vi "Q-Insert.vi"(6 "timeout in ms (-1)":i32=-1, 7 "Queue Type":T1, 8 "error in":errorcluster, 9 "Index":i32, 10 "Read Data":T2, 11 "Q Name":string) -> (0 "error out":errorcluster)   [LabVIEW 2016]
uses:
  PSDAQEG_Task Queue Type.ctl
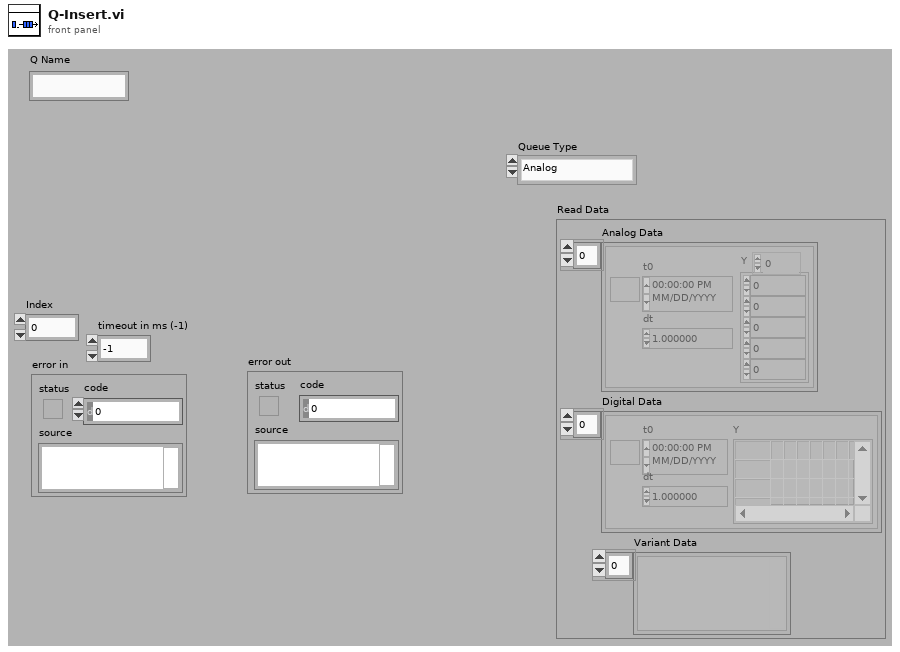
[diagram p1: front panel]
types:
  T1 = typedef "PSDAQEG_Task Queue Type.ctl" = enum16{"Analog", "Digital", "Variant"}
  T2 = cluster{"Analog Data":waveform(dbl)[], "Digital Data":digitalwaveform[], "Variant Data":variant[]}
  T3 = cluster{"Index":i32, "Analog Data":waveform(dbl)[]}
  T4 = cluster{"Index":i32, "Digital Data":digitalwaveform[]}
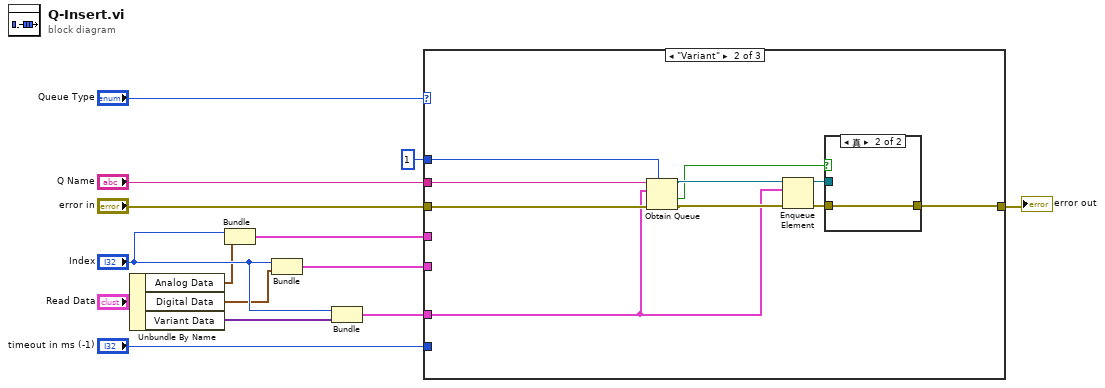
[diagram p0: block diagram]
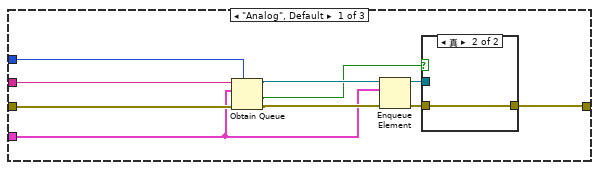
[diagram p2: hidden frame]
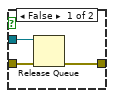
[diagram p3: hidden frame]
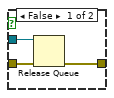
[diagram p4: hidden frame]
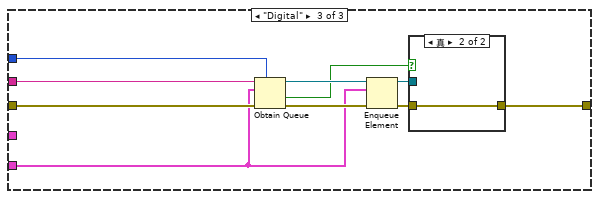
[diagram p5: hidden frame]
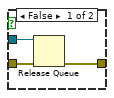
[diagram p6: hidden frame]
diagram:
  n1 = Unbundle By Name("Read Data") -> ("Analog Data"=w1:waveform(dbl)[], "Digital Data"=w3:digitalwaveform[], "Variant Data"=w2:variant[])
  n2 = Bundle("Index"="Index", "Analog Data"=w1) -> (w12:T3)  [unwired: 1 in]
  n3 = Bundle("Index"="Index", "Digital Data"=w3) -> (w13:T4)  [unwired: 1 in]
  n4 = Bundle("Index"="Index", "Variant Data"=w2) -> (w11:cluster{"Index":i32, "Variant Data":variant[]})  [unwired: 1 in]
  n5 = case shown="\"Variant\"" "Queue Type" {
    tunnel: "Q Name" -> [w23 w37 w52]
    tunnel: "error in" -> [w24 w38 w51]
    tunnel: 1 ("Index") -> [w22 w36 w50]
    tunnel: w13 -> [_ _ w43]
    tunnel: [w18 w31 w46] -> w10
    tunnel: w12 -> [w17 _ _]
    tunnel: w11 -> [_ w29 _]
    tunnel: "timeout in ms (-1)" -> [_ _ _]
    frame "Analog", Default {
      n6 = Obtain Queue(max queue size (-1, unlimited)=w22, name (unnamed)=w23, element data type=w17, error in (no error)=w24) -> (queue out=w16:refnum<queue>, created new?=w15:bool, error out=w19:errorcluster)  [unwired: 1 in]
      n7 = Enqueue Element(queue=w16, element=w17, error in (no error)=w19) -> (queue out=w20:refnum<queue>, error out=w21:errorcluster)  [unwired: 1 in, 1 out]
      n8 = case shown="真" w15 {
        tunnel: w20 -> [w27 _]
        tunnel: w21 -> [w26 w28]
        tunnel: [w25 w28] -> w18
        frame False {
          n9 = Release Queue(queue=w27, error in (no error)=w26) -> (error out=w25:errorcluster)  [unwired: 1 in, 2 out]
        }
        frame True {
        }
      }
    }
    frame "Variant" {
      n10 = Obtain Queue(max queue size (-1, unlimited)=w36, name (unnamed)=w37, element data type=w29, error in (no error)=w38) -> (queue out=w32:refnum<queue>, created new?=w30:bool, error out=w33:errorcluster)  [unwired: 1 in]
      n11 = Enqueue Element(queue=w32, element=w29, error in (no error)=w33) -> (queue out=w34:refnum<queue>, error out=w35:errorcluster)  [unwired: 1 in, 1 out]
      n12 = case shown="真" w30 {
        tunnel: w34 -> [w41 _]
        tunnel: w35 -> [w40 w42]
        tunnel: [w39 w42] -> w31
        frame False {
          n13 = Release Queue(queue=w41, error in (no error)=w40) -> (error out=w39:errorcluster)  [unwired: 1 in, 2 out]
        }
        frame True {
        }
      }
    }
    frame "Digital" {
      n14 = Obtain Queue(max queue size (-1, unlimited)=w50, name (unnamed)=w52, element data type=w43, error in (no error)=w51) -> (queue out=w45:refnum<queue>, created new?=w44:bool, error out=w47:errorcluster)  [unwired: 1 in]
      n15 = Enqueue Element(queue=w45, element=w43, error in (no error)=w47) -> (queue out=w48:refnum<queue>, error out=w49:errorcluster)  [unwired: 1 in, 1 out]
      n16 = case shown="真" w44 {
        tunnel: w48 -> [w55 _]
        tunnel: w49 -> [w54 w56]
        tunnel: [w53 w56] -> w46
        frame False {
          n17 = Release Queue(queue=w55, error in (no error)=w54) -> (error out=w53:errorcluster)  [unwired: 1 in, 2 out]
        }
        frame True {
        }
      }
    }
  }
  "error out" <- w10
